vi "Write Control Refs.vi"(10 "Control Refs":T1, 11 "AMS Gas in":refnum<class "AMS Gas.lvclass">) -> (3 "AMS Gas out":refnum<class "AMS Gas.lvclass">)   [LabVIEW 2015, in "AMS UI.lvlib" / "AMS Gas.lvclass"]
uses:
  AMS Gas.lvclass
  Controls/FP Control Refs Cluster.ctl
  Controls/Liquid N Valve Ref Cluster.ctl
  Controls/Main Line Valve Ref Cluster.ctl
  Controls/Sample Valve Refs.ctl
  Controls/Syringe Ctrl Refs.ctl
  AMS Gas.lvclass/AMS Gas.ctl
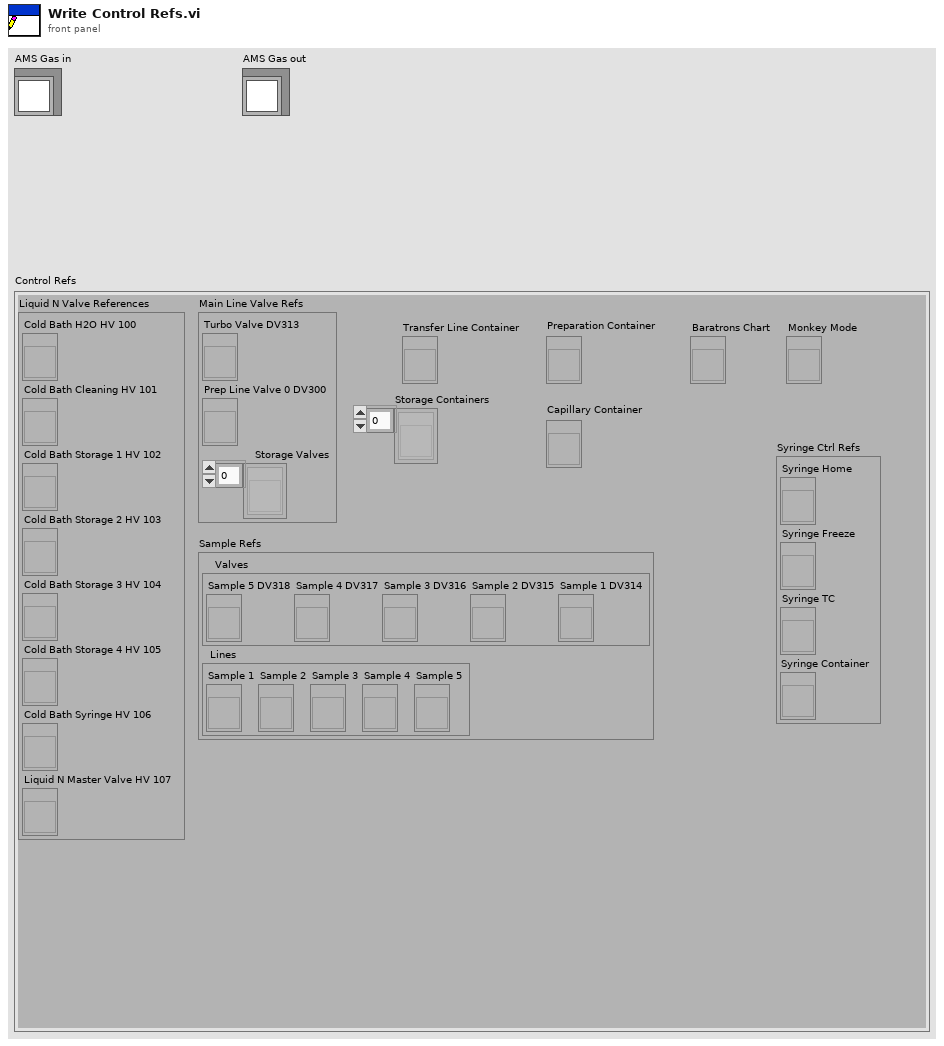
[diagram p1: front panel]
types:
  T1 = typedef "FP Control Refs Cluster.ctl" = cluster{"Liquid N Valve References":T2, "Main Line Valve Refs":T3, "Transfer Line Container":refnum<vi>, "Storage Containers":refnum<vi>[], "Sample Refs":T4, "Syringe Ctrl Refs ":T5, "Baratrons Chart":refnum<vi>, "Capillary Container":refnum<vi>, "Preparation Container":refnum<vi>, "Monkey Mode":refnum<vi>}
  T2 = typedef "Liquid N Valve Ref Cluster.ctl" = cluster{"Cold Bath H2O HV 100":refnum<vi>, "Cold Bath Cleaning HV 101":refnum<vi>, "Cold Bath Storage 1 HV 102":refnum<vi>, "Cold Bath Storage 2 HV 103":refnum<vi>, "Cold Bath Storage 3 HV 104":refnum<vi>, "Cold Bath Storage 4 HV 105":refnum<vi>, "Cold Bath Syringe HV 106":refnum<vi>, "Liquid N Master Valve HV 107":refnum<vi>}
  T3 = typedef "Main Line Valve Ref Cluster.ctl" = cluster{"Turbo Valve DV313":refnum<vi>, "Prep Line Valve 0 DV300":refnum<vi>, "Storage Valves":refnum<vi>[]}
  T4 = typedef "Sample Valve Refs.ctl" = cluster{"Valves":cluster{"Sample 5 DV318":refnum<vi>, "Sample 4 DV317":refnum<vi>, "Sample 3 DV316":refnum<vi>, "Sample 2 DV315":refnum<vi>, "Sample 1 DV314":refnum<vi>}, "Lines":cluster{"Sample 1":refnum<vi>, "Sample 2":refnum<vi>, "Sample 3":refnum<vi>, "Sample 4":refnum<vi>, "Sample 5":refnum<vi>}}
  T5 = typedef "Syringe Ctrl Refs.ctl" = cluster{"Syringe Home":refnum<vi>, "Syringe Freeze":refnum<vi>, "Syringe TC":refnum<vi>, "Syringe Container":refnum<vi>}
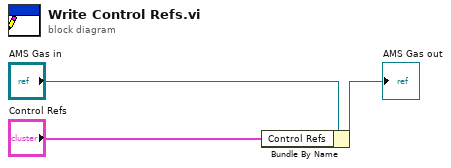
[diagram p0: block diagram]
diagram:
  n1 = Bundle By Name(cluster="AMS Gas in", "Control Refs"="Control Refs") -> (→"AMS Gas out":refnum<class "AMS Gas.lvclass">)
